vi "Source Open.vi"(8 "error in":errorcluster, 11 "src in":T1={"type"=enum."Tektronix AFG3101C", "idn"="", "afg"={"VISA"="", "const"=0.0, "gen DC"=FALSE, "ext ref"=FALSE}, "cDAQ dds"={"device"="", "channels"=[], "mclk source"="", "mclk [Hz]"=0.0, "fs [Hz]"=0.0, "block [s]"=0.0, "buf [s]"=0.0, "task"="", "cmd queue"=refnum, "proc ref"=refnum, "smpl clock out"="/cDAQ3/PFI0", "export smpl clock"=FALSE, "DC ofs [V]"=[], "timebase source"="", "timebase mode"=enum."Local", "dither"=enum."Disabled", "dither level"=0.0, "phase [rad]"=[]}, "gain [V/A]"=1.0, "F5xxx session"={"VISA"="", "mode"=enum."AC voltage", "Earth on"=FALSE, "Ext ref lock"=FALSE}, "t3awg"={"VISA"="", "use ext ref"=FALSE, "ext ref [Hz]"=0.0, "load Z"=enum."High Z", "ramdac max n"=0, "noise dither [V]"=0.0, "t3awg fs rules"=[], "channels"=0, "ramdac min n"=0, "channel list"=[], "gen resl [Vpp]"=0.0, "wave data format"=enum."Binary"}} {"t3awg"."t3awg fs rules"."fs-step [Hz]" format="%#_6p"; "t3awg"."t3awg fs rules"."fs-max [Hz]" format="%#_6p"; "t3awg"."t3awg fs rules"."for f0 <" format="%#_6p"; "t3awg"."t3awg fs rules"."fs-min [Hz]" format="%#_6p"; "cDAQ dds"."channels" min=0 step=1}) -> (0 "error out":errorcluster, 2 "idn string":string, 3 "src out":T1={"type"=enum."Tektronix AFG3101C", "idn"="", "afg"={"VISA"="", "const"=0.0, "gen DC"=FALSE, "ext ref"=FALSE}, "cDAQ dds"={"device"="", "channels"=[], "mclk source"="", "mclk [Hz]"=0.0, "fs [Hz]"=0.0, "block [s]"=0.0, "buf [s]"=0.0, "task"="", "cmd queue"=refnum, "proc ref"=refnum, "smpl clock out"="/cDAQ3/PFI0", "export smpl clock"=FALSE, "DC ofs [V]"=[], "timebase source"="", "timebase mode"=enum."Local", "dither"=enum."Disabled", "dither level"=0.0, "phase [rad]"=[]}, "gain [V/A]"=1.0, "F5xxx session"={"VISA"="", "mode"=enum."AC voltage", "Earth on"=FALSE, "Ext ref lock"=FALSE}, "t3awg"={"VISA"="", "use ext ref"=FALSE, "ext ref [Hz]"=0.0, "load Z"=enum."High Z", "ramdac max n"=0, "noise dither [V]"=0.0, "t3awg fs rules"=[], "channels"=0, "ramdac min n"=0, "channel list"=[], "gen resl [Vpp]"=0.0, "wave data format"=enum."Binary"}} {"t3awg"."t3awg fs rules"."fs-step [Hz]" format="%#_6p"; "t3awg"."t3awg fs rules"."fs-max [Hz]" format="%#_6p"; "t3awg"."t3awg fs rules"."for f0 <" format="%#_6p"; "t3awg"."t3awg fs rules"."fs-min [Hz]" format="%#_6p"; "cDAQ dds"."channels" min=0 step=1})   [LabVIEW 2020]
doc: "Open source."
uses:
  Source Session.ctl
  Source Type.ctl
  drivers/AFG3101C/AFG3101C Session.ctl
  drivers/cDAQ DDS/cDAQ DDS Session.ctl
  drivers/cDAQ DDS/cDAQ DDS Setup.ctl
  drivers/cDAQ DDS/cDAQ DDS Timebase Mode.ctl
  drivers/cDAQ DDS/cDAQ DDS Dither.ctl
  drivers/Fluke 5XXX/top_lev/F5xxx_session.ctl
  drivers/Fluke 5XXX/top_lev/F5xxx_output_mode.ctl
  drivers/T3AWG3K/toplevel/T3AWG Session.ctl
  drivers/T3AWG3K/toplevel/T3AWG Load Z.ctl
  drivers/T3AWG3K/toplevel/fgen_ramdac_fs_rules.ctl
  drivers/T3AWG3K/toplevel/T3AWG Channel.ctl
  drivers/AFG3101C/Tektronix AFG 3000 Series.lvlib
  <vilib>/ErrorRing/Error Ring.xnode
  <vilib>/Utility/error.llb/Error Cluster From Error Code.vi
  drivers/Agilent 33XXX Series/Agilent 33XXX Series.lvlib
  drivers/T3AWG3K/Active Technologies AWG3000.lvlib
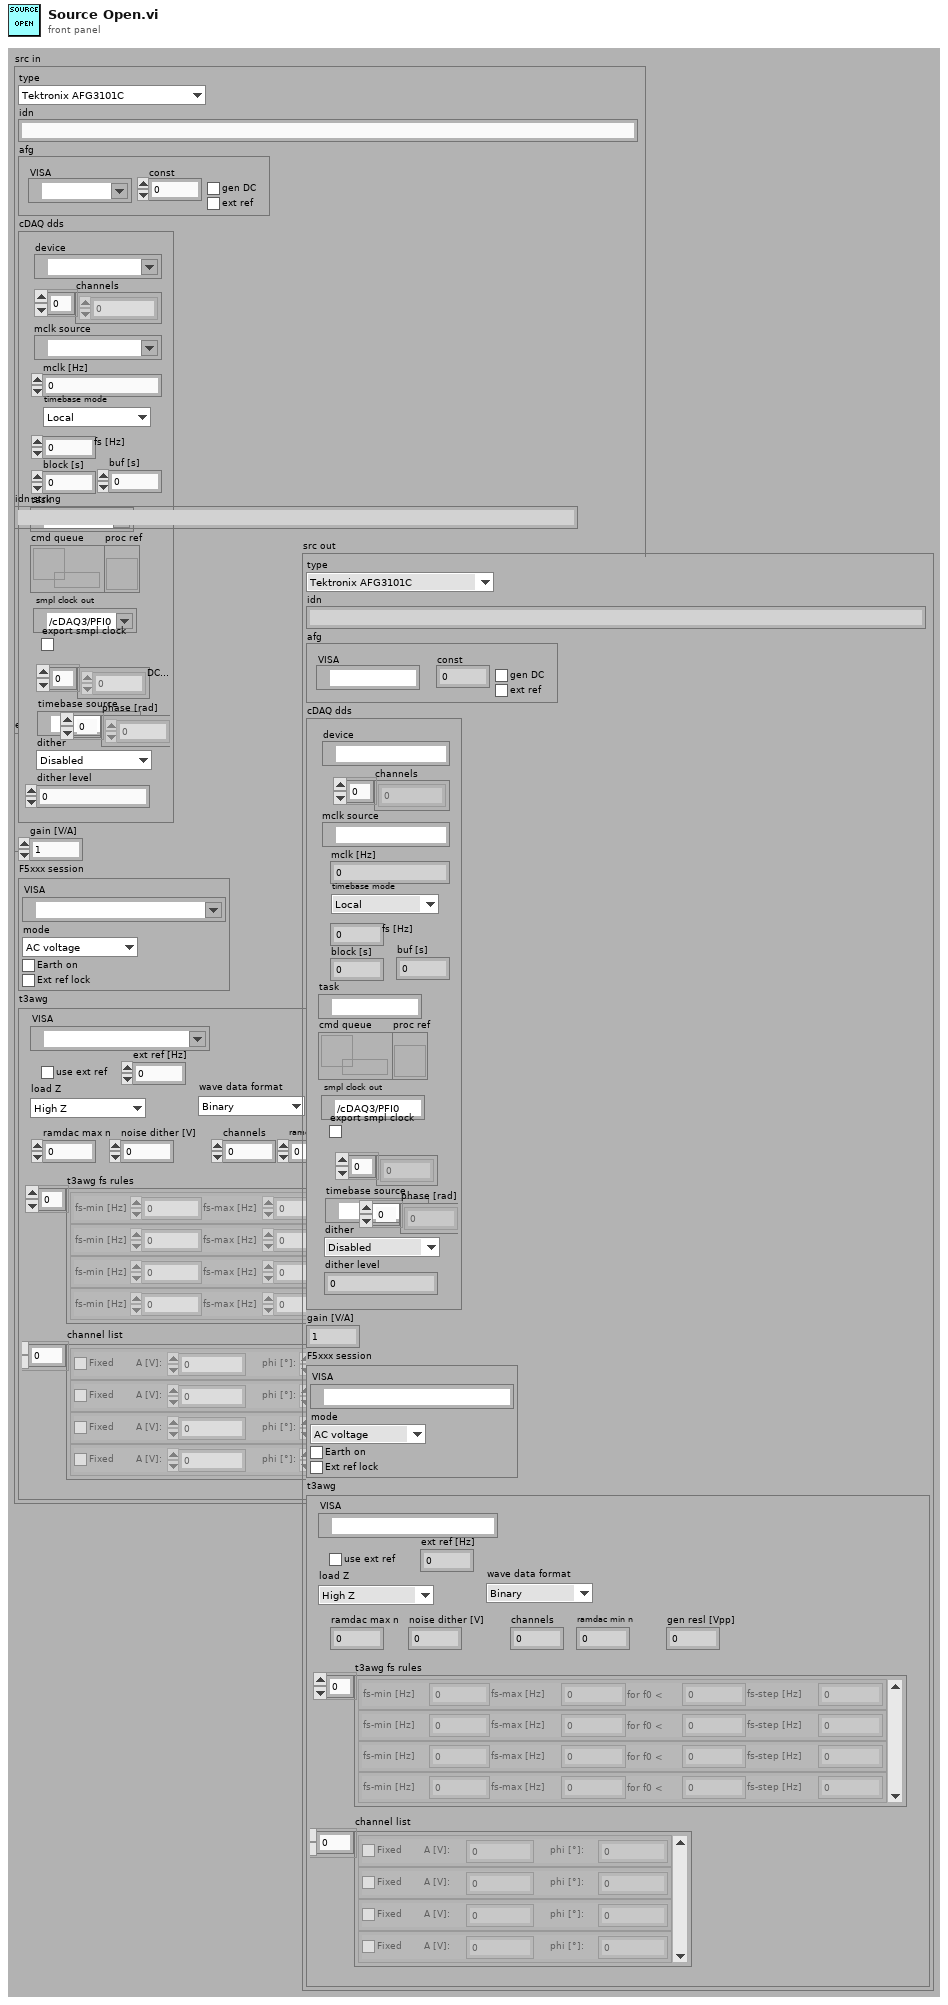
[diagram p1: front panel]
types:
  T1 = typedef "Source Session.ctl" = cluster{"type":T2, "idn":string, "afg":T3, "cDAQ dds":T4, "gain [V/A]":dbl, "F5xxx session":T7, "t3awg":T9}
  T2 = typedef "Source Type.ctl" = enum16{"Tektronix AFG3101C", "cDAQ DAC", "Fluke 5xxx", "Datron 4xxx", "Agilent 33120A", "R&S SMT", "Teledyne LeCroy T3AWG", "dummy"}
  T3 = typedef "AFG3101C Session.ctl" = cluster{"VISA":refnum<visa-resource-name>, "const":dbl, "gen DC":bool, "ext ref":bool}
  T4 = typedef "cDAQ DDS Session.ctl" = cluster{"device":tag, "channels":i32[], "mclk source":tag, "mclk [Hz]":dbl, "fs [Hz]":dbl, "block [s]":dbl, "buf [s]":dbl, "task":refnum<k21>, "cmd queue":refnum<queue>, "proc ref":refnum<vi>, "smpl clock out":tag, "export smpl clock":bool, "DC ofs [V]":dbl[], "timebase source":tag, "timebase mode":T5, "dither":T6, "dither level":dbl, "phase [rad]":dbl[]}
  T5 = typedef "cDAQ DDS Timebase Mode.ctl" = enum16{"Local", "Take from ADC (e.g. NI 9238)", "Other source"}
  T6 = typedef "cDAQ DDS Dither.ctl" = enum16{"Disabled", "Gaussian"}
  T7 = typedef "F5xxx_session.ctl" = cluster{"VISA":refnum<visa-resource-name>, "mode":T8, "Earth on":bool, "Ext ref lock":bool}
  T8 = typedef "F5xxx_output_mode.ctl" = enum16{"AC voltage", "AC current"}
  T9 = typedef "Active Technologies AWG3000.lvlib/T3AWG Session.ctl" = cluster{"VISA":refnum<visa-resource-name>, "use ext ref":bool, "ext ref [Hz]":dbl, "load Z":T10, "ramdac max n":i32, "noise dither [V]":dbl, "t3awg fs rules":T11[], "channels":i32, "ramdac min n":i32, "channel list":T12[], "gen resl [Vpp]":dbl, "wave data format":T13}
  T10 = typedef "Active Technologies AWG3000.lvlib/T3AWG Load Z.ctl" = enum16{"High Z", "50 Ohm"}
  T11 = typedef "Active Technologies AWG3000.lvlib/fgen_ramdac_fs_rules.ctl" = cluster{"fs-min [Hz]":dbl, "fs-max [Hz]":dbl, "for f0 < ":dbl, "fs-step [Hz]":dbl}
  T12 = typedef "Active Technologies AWG3000.lvlib/T3AWG Channel.ctl" = cluster{"Fixed":bool, "A [V]:":dbl, "phi [°]:":dbl}
  T13 = typedef "Active Technologies AWG3000.lvlib/T3AWG Wave Format" = enum16{"Text", "Binary"}
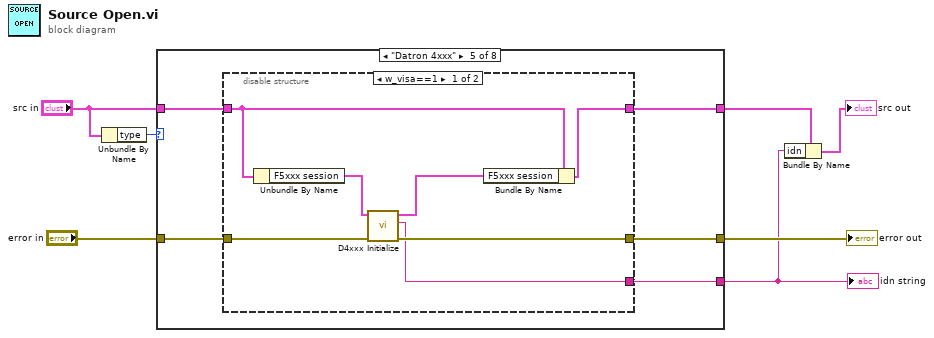
[diagram p0: block diagram]
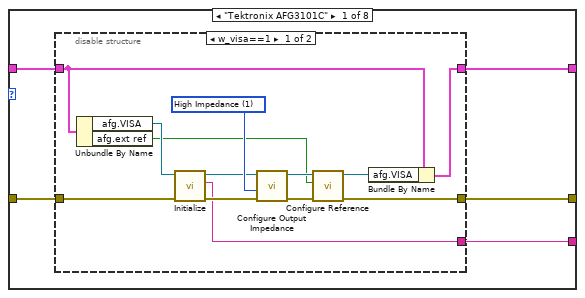
[diagram p2: hidden frame]
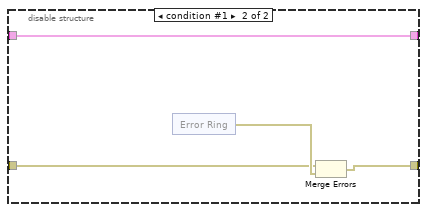
[diagram p3: hidden frame]
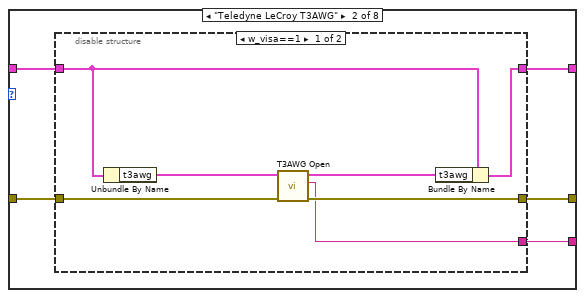
[diagram p4: hidden frame]
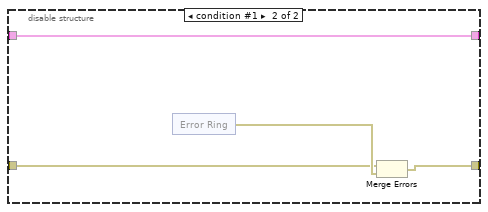
[diagram p5: hidden frame]
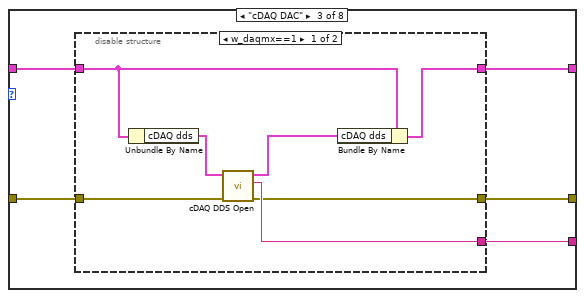
[diagram p6: hidden frame]
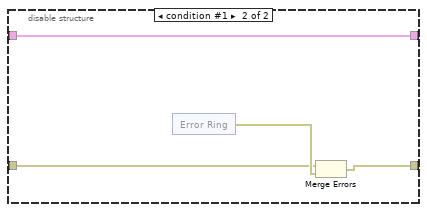
[diagram p7: hidden frame]
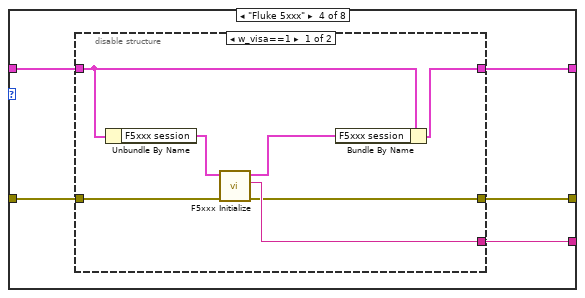
[diagram p8: hidden frame]
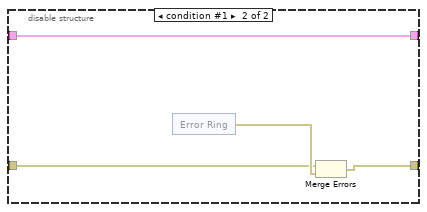
[diagram p9: hidden frame]
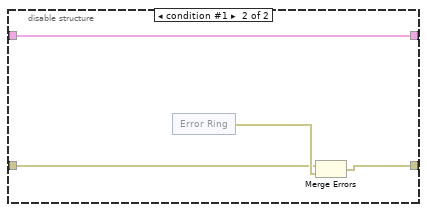
[diagram p10: hidden frame]
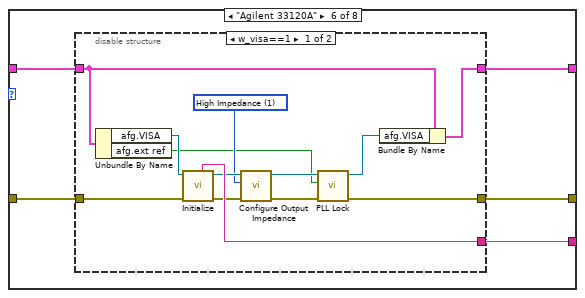
[diagram p11: hidden frame]
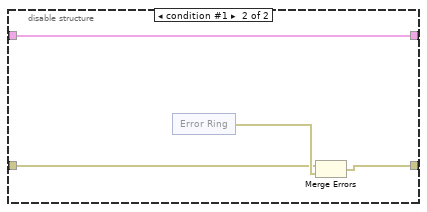
[diagram p12: hidden frame]
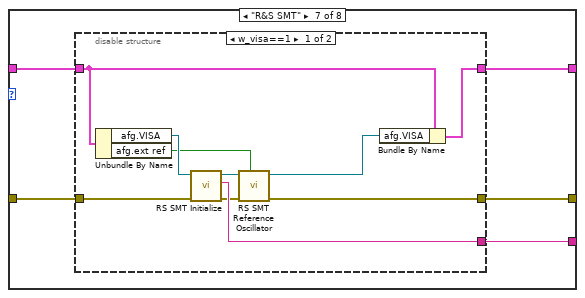
[diagram p13: hidden frame]
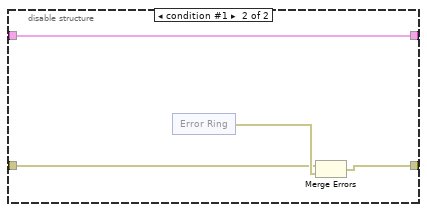
[diagram p14: hidden frame]
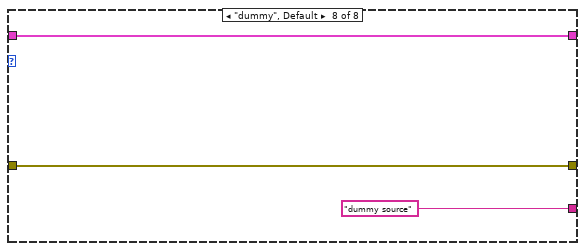
[diagram p15: hidden frame]
diagram:
  n1 = Unbundle By Name("src in") -> ("type"=w6:T2)
  n2 = case shown="\"Datron 4xxx\"" w6 {
    tunnel: "src in" -> [w12 w39 w59 w80 w101 w122 w149 w172]
    tunnel: "error in" -> [w8 w35 w60 w81 w102 w123 w150 w171]
    tunnel: [w10 w37 w57 w78 w99 w120 w147 w171] -> w4
    tunnel: [w11 w38 w56 w77 w98 w119 w146 w172] -> w3
    tunnel: [w9 w36 w58 w79 w100 w121 w148 "dummy source" ("idn string")] -> w1
    frame "Tektronix AFG3101C" {
      n3 = disable-structure shown="w_visa==1" {
        disable-tunnel: w8 -> [w18 w27]
        disable-tunnel: w12 -> [w21 w29]
        disable-tunnel: [w14 w26] -> w10
        disable-tunnel: [w20 w29] -> w11
        disable-tunnel: [w19 _] -> w9
        frame condition #0 (active) {
          w25 = u16 1 items=["50 Ohm", "High Impedance", "Customized"] ("Impedance (0: 50 Ohm)")
          n4 = Unbundle By Name(w21) -> ("afg.VISA"=w22:refnum<visa-resource-name>, "afg.ext ref"=w13:bool)
          n5 = call "Initialize.vi"("error in (no error)"=w18, "VISA resource name"=w22) -> ("error out"=w23:errorcluster, "idn string"=w19:string, "VISA resource name out"=w24:refnum<visa-resource-name>)  [unwired: 7 in]
          n6 = call "Configure Output Impedance.vi"("error in (no error)"=w23, "Impedance (0: 50 Ohm)"=w25, "VISA resource name"=w24) -> ("error out"=w17:errorcluster, "VISA resource name out"=w16:refnum<visa-resource-name>)  [unwired: 7 in]
          n7 = call "Configure Reference.vi"("error in (no error)"=w17, "external clock"=w13, "VISA resource name"=w16) -> ("error out"=w14:errorcluster, "VISA resource name out"=w15:refnum<visa-resource-name>)  [unwired: 7 in]
          n8 = Bundle By Name(cluster=w21, "afg.VISA"=w15) -> (w20:T1)
        }
        frame condition #1 {
          n9 = xnode "Error Ring"() -> ("error out"=w28:errorcluster)
          n10 = Merge Errors(w27, w28) -> (w26:errorcluster)
        }
      }
    }
    frame "Teledyne LeCroy T3AWG" {
      n11 = disable-structure shown="w_visa==1" {
        disable-tunnel: w35 -> [w43 w48]
        disable-tunnel: w39 -> [w46 w50]
        disable-tunnel: [w41 w47] -> w37
        disable-tunnel: [w45 w50] -> w38
        disable-tunnel: [w40 _] -> w36
        frame condition #0 (active) {
          n12 = Unbundle By Name(w46) -> ("t3awg"=w44:T9)
          n13 = call "T3AWG Open.vi"("error in (no error)"=w43, "t3awg"=w44) -> ("error out"=w41:errorcluster, "idn string"=w40:string, "t3awg out"=w42:T9)  [unwired: 7 in]
          n14 = Bundle By Name(cluster=w46, "t3awg"=w42) -> (w45:T1)
        }
        frame condition #1 {
          n15 = xnode "Error Ring"() -> ("error out"=w49:errorcluster)
          n16 = Merge Errors(w48, w49) -> (w47:errorcluster)
        }
      }
    }
    frame "cDAQ DAC" {
      n17 = disable-structure shown="w_daqmx==1" {
        disable-tunnel: w60 -> [w67 w69]
        disable-tunnel: w59 -> [w65 w71]
        disable-tunnel: [w63 _] -> w58
        disable-tunnel: [w62 w68] -> w57
        disable-tunnel: [w61 w71] -> w56
        frame condition #0 (active) {
          n18 = Unbundle By Name(w65) -> ("cDAQ dds"=w66:T4)
          n19 = call "cDAQ DDS Open.vi"("error in"=w67, "session in"=w66) -> ("error out"=w62:errorcluster, "idn string"=w63:string, "session out"=w64:T4)  [unwired: 7 in]
          n20 = Bundle By Name(cluster=w65, "cDAQ dds"=w64) -> (w61:T1)
        }
        frame condition #1 {
          n21 = xnode "Error Ring"() -> ("error out"=w70:errorcluster)
          n22 = Merge Errors(w69, w70) -> (w68:errorcluster)
        }
      }
    }
    frame "Fluke 5xxx" {
      n23 = disable-structure shown="w_visa==1" {
        disable-tunnel: w81 -> [w88 w90]
        disable-tunnel: w80 -> [w86 w92]
        disable-tunnel: [w84 _] -> w79
        disable-tunnel: [w83 w89] -> w78
        disable-tunnel: [w82 w92] -> w77
        frame condition #0 (active) {
          n24 = Unbundle By Name(w86) -> ("F5xxx session"=w87:T7)
          n25 = call "F5xxx Initialize.vi"("error in (no error)"=w88, "session in"=w87) -> ("error out"=w83:errorcluster, "idn string"=w84:string, "session out"=w85:T7)  [unwired: 7 in]
          n26 = Bundle By Name(cluster=w86, "F5xxx session"=w85) -> (w82:T1)
        }
        frame condition #1 {
          n27 = xnode "Error Ring"() -> ("error out"=w91:errorcluster)
          n28 = Merge Errors(w90, w91) -> (w89:errorcluster)
        }
      }
    }
    frame "Datron 4xxx" {
      n29 = disable-structure shown="w_visa==1" {
        disable-tunnel: w102 -> [w109 w111]
        disable-tunnel: w101 -> [w108 w113]
        disable-tunnel: [w103 _] -> w100
        disable-tunnel: [w106 w110] -> w99
        disable-tunnel: [w105 w113] -> w98
        frame condition #0 (active) {
          n30 = Unbundle By Name(w108) -> ("F5xxx session"=w104:T7)
          n31 = call "D4xxx Initialize.vi"("error in (no error)"=w109, "session in"=w104) -> ("error out"=w106:errorcluster, "idn string"=w103:string, "session out"=w107:T7)  [unwired: 7 in]
          n32 = Bundle By Name(cluster=w108, "F5xxx session"=w107) -> (w105:T1)
        }
        frame condition #1 {
          n33 = xnode "Error Ring"() -> ("error out"=w112:errorcluster)
          n34 = Merge Errors(w111, w112) -> (w110:errorcluster)
        }
      }
    }
    frame "Agilent 33120A" {
      n35 = disable-structure shown="w_visa==1" {
        disable-tunnel: w123 -> [w134 w138]
        disable-tunnel: w122 -> [w136 w140]
        disable-tunnel: [w132 _] -> w121
        disable-tunnel: [w127 w137] -> w120
        disable-tunnel: [w135 w140] -> w119
        frame condition #0 (active) {
          w129 = u16 1 items=["50 Ohms", "High Impedance", "User Defined"] ("Impedance (0: 50 Ohms)")
          n36 = Unbundle By Name(w136) -> ("afg.VISA"=w133:refnum<visa-resource-name>, "afg.ext ref"=w124:bool)
          n37 = call "Initialize.vi"("error in (no error)"=w134, "VISA resource name"=w133) -> ("error out"=w131:errorcluster, "VISA resource name out"=w130:refnum<visa-resource-name>, "ID"=w132:string)  [unwired: 7 in]
          n38 = call "Configure Output Impedance.vi"("error in (no error)"=w131, "Impedance (0: 50 Ohms)"=w129, "VISA resource name"=w130) -> ("error out"=w128:errorcluster, "VISA resource name out"=w125:refnum<visa-resource-name>)  [unwired: 7 in]
          n39 = call "PLL Lock.vi"("error in (no error)"=w128, "PLL lock  (T: Enable)"=w124, "VISA resource name"=w125) -> ("error out"=w127:errorcluster, "VISA resource name out"=w126:refnum<visa-resource-name>)  [unwired: 7 in]
          n40 = Bundle By Name(cluster=w136, "afg.VISA"=w126) -> (w135:T1)
        }
        frame condition #1 {
          n41 = xnode "Error Ring"() -> ("error out"=w139:errorcluster)
          n42 = Merge Errors(w138, w139) -> (w137:errorcluster)
        }
      }
    }
    frame "R&S SMT" {
      n43 = disable-structure shown="w_visa==1" {
        disable-tunnel: w150 -> [w158 w162]
        disable-tunnel: w149 -> [w160 w164]
        disable-tunnel: [w156 _] -> w148
        disable-tunnel: [w152 w161] -> w147
        disable-tunnel: [w159 w164] -> w146
        frame condition #0 (active) {
          n44 = Unbundle By Name(w160) -> ("afg.VISA"=w157:refnum<visa-resource-name>, "afg.ext ref"=w153:bool)
          n45 = call "RS SMT Initialize.vi"("error in (no error)"=w158, "Instr. Descriptor (GPIB::28)"=w157) -> ("error out"=w155:errorcluster, "idn string"=w156:string, "VISA session"=w154:refnum<visa-resource-name>)  [unwired: 7 in]
          n46 = call "RS SMT Reference Oscillator.vi"("Ref Source (F:Int)"=w153, "error in (no error)"=w155, "VISA session"=w154) -> ("error out"=w152:errorcluster, "dup VISA session"=w151:refnum<visa-resource-name>)  [unwired: 7 in]
          n47 = Bundle By Name(cluster=w160, "afg.VISA"=w151) -> (w159:T1)
        }
        frame condition #1 {
          n48 = xnode "Error Ring"() -> ("error out"=w163:errorcluster)
          n49 = Merge Errors(w162, w163) -> (w161:errorcluster)
        }
      }
    }
    frame "dummy", Default {
    }
  }
  "error out" <- w4
  "idn string" <- w1
  n50 = Bundle By Name(cluster=w3, "idn"=w1) -> (→"src out":T1)
